vi "UI_Initialize.vi"(8 "error in (no error)":errorcluster, 10 "UI_Object":T1, 11 "PLC_Module in":refnum<class "PLC_Module.lvclass">) -> (0 "error out":errorcluster, 3 "PLC_Module out":refnum<class "PLC_Module.lvclass">)   [LabVIEW 2025, in "PLC_Module.lvlib" / "PLC_Module.lvclass"]
uses:
  PLC_Module.lvclass
  UI_Object.ctl
  PLC_Module.lvclass/PLC_Module.ctl
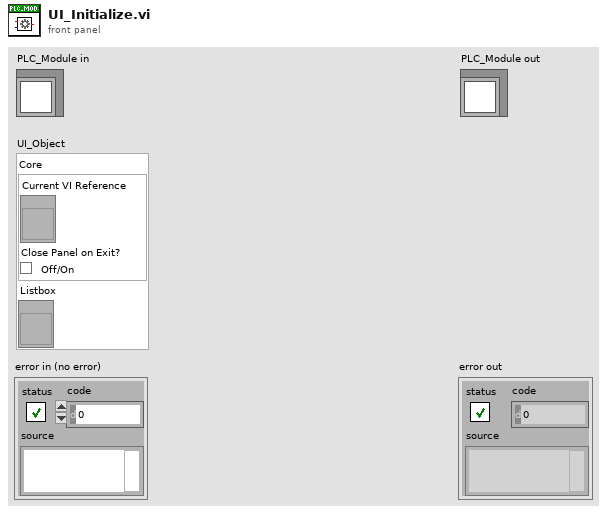
[diagram p1: front panel]
types:
  T1 = typedef "PLC_Module.lvlib/PLC_Module.lvclass/UI_Object.ctl" = cluster{"Core":cluster{"Current VI Reference":refnum<vi>, "Close Panel on Exit?":bool}, "Listbox":refnum<vi>}
  T2 = typedef "PLC_Module.lvlib/PLC_Module.lvclass/PLC_Type.ctl" = enum16{"Simulated_PLC", "SIMATIC_S7"}
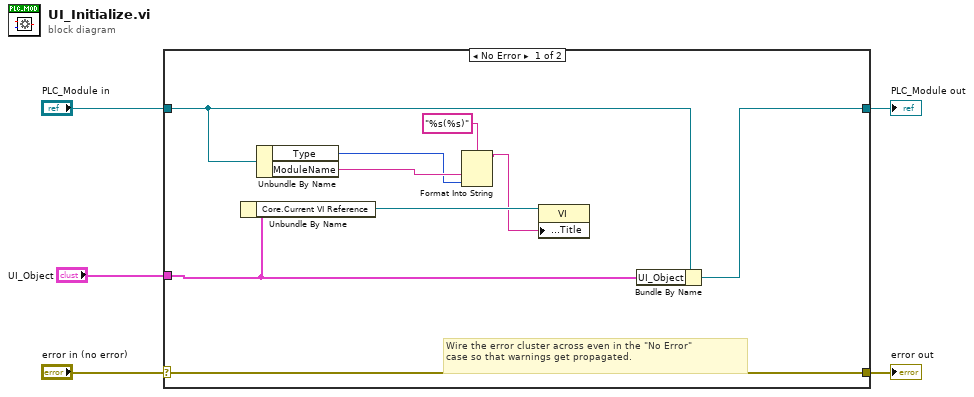
[diagram p0: block diagram]
diagram:
  n1 = case shown="No Error" "error in (no error)" {
    selector: "error in (no error)" -> [w14 w16]
    tunnel: [w14 w16] -> w4
    tunnel: [w12 w15] -> w2
    tunnel: "PLC_Module in" -> [w13 w15]
    tunnel: "UI_Object" -> [w11 _]
    frame No Error {
      # "Wire the error cluster across even in the \"No Error\"\ncase so that warnings get propagated."
      n2 = Unbundle By Name(w11) -> ("Core.Current VI Reference"=w10:refnum<vi>)
      n3 = Unbundle By Name(w13) -> ("Type"=w7:T2, "ModuleName"=w8:string)
      n4 = Format Into String(format string="%s(%s)", w8, w7) -> (resulting string=w6:string)  [unwired: 2 in, 1 out]
      n5 = property class="VI"(reference=w10, "Front Panel.Title"=w6) -> ()  [unwired: 1 in, 2 out]
      n6 = Bundle By Name(cluster=w13, "UI_Object"=w11) -> (w12:refnum<class "PLC_Module.lvclass">)
    }
    frame Error {
    }
  }
  "error out" <- w4
  "PLC_Module out" <- w2
